vi "Create Header.vi"(8 "error in (no error)":errorcluster, 11 "Header Parameters":T1[](array[typedef])) -> (0 "error out":errorcluster, 3 "Header":string)   [LabVIEW 2011, in "i3-oauth.lvlib"]
doc: "Use this template to build a VI to use as a subVI."
uses:
  i3-oauth.lvlib
  Controls/Name-Value Pair.ctl
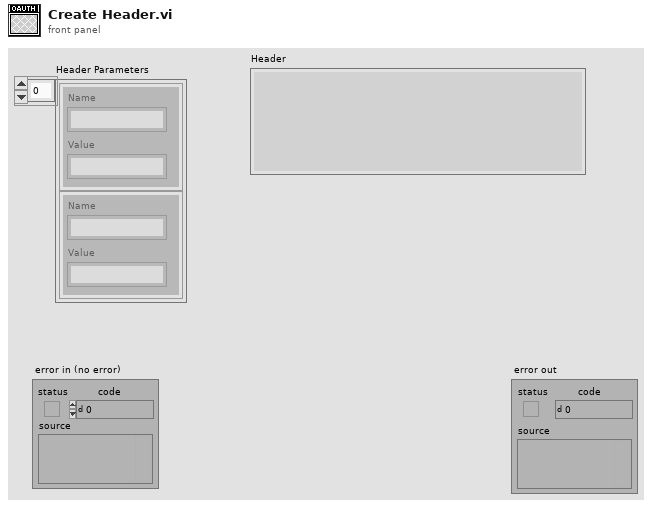
[diagram p1: front panel]
types:
  T1 = typedef "i3-oauth.lvlib/Name-Value Pair.ctl" = cluster{"Name":string, "Value":string}
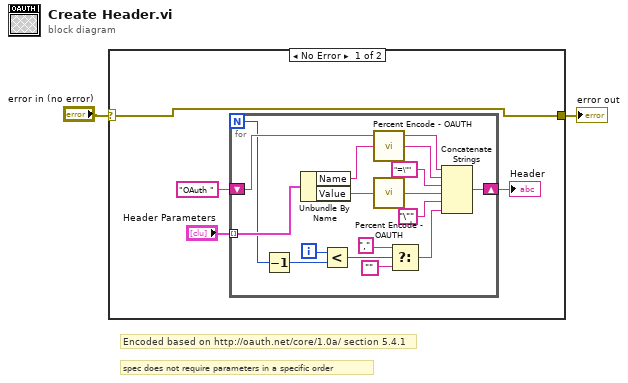
[diagram p0: block diagram]
diagram:
  # "spec does not require parameters in a specific order"
  # "Encoded based on http://oauth.net/core/1.0a/ section 5.4.1"
  n1 = case shown="No Error" "error in (no error)" {
    selector: "error in (no error)" -> [w3 w23]
    tunnel: [w3 w23] -> w1
    frame No Error {
      n2 = for {
        N -> [w17]
        shift-right: [w19] -> w5
        shift-left: "OAuth " -> [w21]
        tunnel: "Header Parameters" -> [w22] mode=indexing
        i -> [w18]
        n3 = Decrement(x=w17) -> (x-1=w16:i32)
        n4 = Unbundle By Name(w22) -> ("Name"=w10:string, "Value"=w8:string)
        n5 = Less?(x=w18, y=w16) -> (x < y?=w14:bool)
        n6 = call "Percent Encode - OAUTH.vi"("unescaped string in"=w10) -> ("escaped string out"=w9:string)
        n7 = call "Percent Encode - OAUTH.vi"("unescaped string in"=w8) -> ("escaped string out"=w7:string)
        n8 = Select(t=",", s=w14, f="") -> (s? t:f=w11:string)
        n9 = Concatenate Strings(w21, w9, "=\"" ("string"), w7, "\"" ("string"), w11) -> (w19:string)
      }
      "Header" <- w5
    }
    frame Error {
    }
  }
  "error out" <- w1
